vi "Lift To Inch.vi"(7 "Speed":dbl=1.0, 11 "Inches to move":dbl) -> (2 "Done":bool)   [LabVIEW 2014]
uses:
  Begin/Global Variables.vi
  <vilib>/Rock Robotics/Network Tables/SD Write Boolean.vi
  Begin/Global RefNums.vi
  <vilib>/Rock Robotics/Network Tables/SD Write Number.vi
panel:
  in  "slave offset":dbl=600.0
  in  "right PID gains":T1={"proportional gain (Kc)"=0.00225, "integral time (Ti, min)"=0.0, "derivative time (Td, min)"=0.0003} {"derivative time (Td, min)" format="%.4f"; "integral time (Ti, min)" format="%.6f"; "proportional gain (Kc)" format="%.5f"}
  in  "left PID gains":T2={"proportional gain (Kc)"=0.003, "integral time (Ti, min)"=0.0, "derivative time (Td, min)"=0.0005} {"derivative time (Td, min)" format="%.10f"; "proportional gain (Kc)" format="%.5f"}
  in  "Output Range":cluster{"output high":dbl, "output low":dbl}={"output high"=0.5, "output low"=-0.5} {"output low" format="%.2f"; "output high" format="%.2f"}
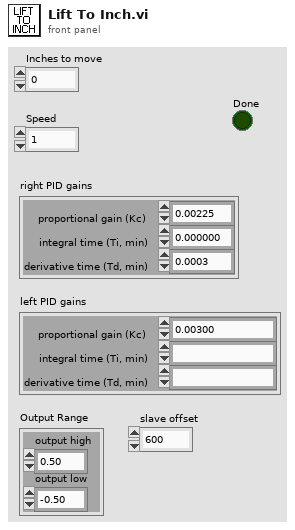
[diagram p1: front panel]
types:
  T1 = cluster{"proportional gain (Kc)":dbl, "integral time (Ti, min)":dbl, "derivative time (Td, min)":dbl}
  T2 = cluster{"proportional gain (Kc)":dbl, "integral time (Ti, min)":fxp<+/-,64,32>, "derivative time (Td, min)":dbl}
  T3 = typedef "WPI_EncoderDevRef.ctl" = cluster{"DevStatus":errorcluster, "EncoderIndex":T4, "CounterIndex":T5, "DistancePerCount":dbl, "Decoding Type":T6}
  T4 = typedef "FPGA_EncoderIdx.ctl" = enum8{"Enc 0", "Enc 1", "Enc 2", "Enc 3", "Enc 4", "Enc 5", "Enc 6", "Enc 7", "Invalid"}
  T5 = typedef "FPGA_CounterCtrSystemIndex.ctl" = enum8{"Ctr 0", "Ctr 1", "Ctr 2", "Ctr 3", "Ctr 4", "Ctr 5", "Ctr 6", "Ctr 7", "Invalid"}
  T6 = typedef "WPI_EncoderType.ctl" = enum16{"1x", "2x", "4x"}
  T7 = typedef "WPI_MotorControlDeviceRef.ctl" = cluster{"DeviceStatus":errorcluster, "Type":T8, "PWM":cluster{"Controller":T9, "PWM Channel":T10, "DeadBand":T11}, "CAN":cluster{"Device Number":u8, "Control Mode":T12, "Semaphore":T13, "Max Vout":dbl, "TalonSRX Control Mode":T14}, "Invert":bool, "TransformRef":T15, "InvTransformRef":T15}
  T8 = typedef "WPI_MotorControlType.ctl" = enum16{"PWM", "CAN", "CANTalonSRX"}
  T9 = typedef "FPGA_TypedefDigitalModule.ctl" = enum16{"Controller 1"}
  T10 = typedef "FPGA_DIOPWMChannel.ctl" = enum8{"PWM 0", "PWM 1", "PWM 2", "PWM 3", "PWM 4", "PWM 5", "PWM 6", "PWM 7", "PWM 8", "PWM 9", "PWM MXP 0", "PWM MXP 1", "PWM MXP 2", "PWM MXP 3", "PWM MXP 4", "PWM MXP 5", "PWM MXP 6", "PWM MXP 7", "PWM MXP 8", "PWM MXP 9", "Invalid"}
  T11 = typedef "WPI_PWMDeadband.ctl" = cluster{"Name":string, "maxPositivePwm":i32, "minPositivePwm":i32, "centerPwm":i32, "maxNegativePwm":i32, "minNegativePwm":i32, "angularRange":u16}
  T12 = typedef "WPI_CANJaguar_ControlMode.ctl" = enum8{"Percent VBus", "Current", "Speed", "Position", "Voltage"}
  T13 = typedef "Semaphore RefNum" = refnum<k1>
  T14 = typedef "WPI_CANTalonSRX_APIControlMode.ctl" = enum8{"Percent VBus", "Speed", "Position", "Slave", "Unchanged / Invalid"}
  T15 = typedef "WPI_PWMTransform_ConPane.ctl" = refnum<vi>
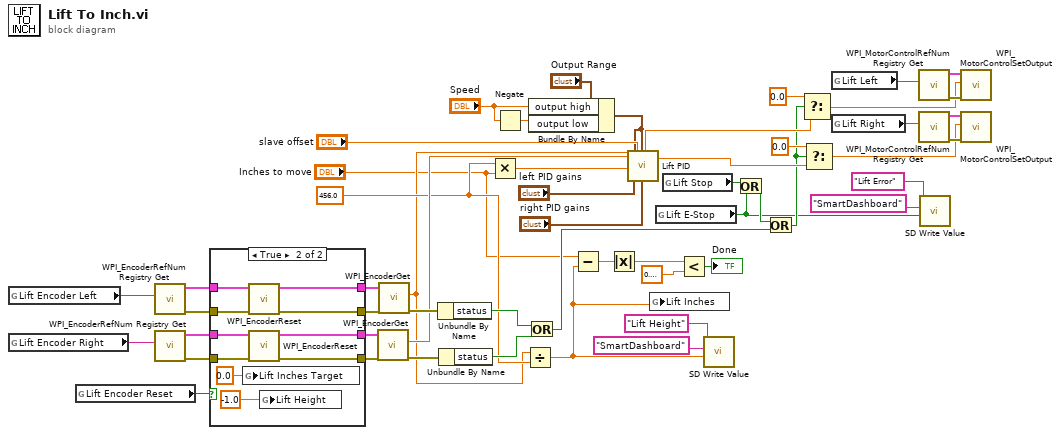
[diagram p0: block diagram]
diagram:
  w4 = 456.0 ("y")
  n1 = global read "Global RefNums.vi" "Lift Encoder Left"() -> (w14:string)
  n2 = global read "Global RefNums.vi" "Lift Encoder Right"() -> (w13:string)
  n3 = global read "Global Variables.vi" "Lift Encoder Reset"() -> (w3:bool)
  n4 = call <vilib>:"WPI_EncoderRefNum Registry Get.vi"("refnum name"=w14) -> ("error out"=w48:errorcluster, "EncoderDevRef"=w47:T3)  [unwired: 9 in]
  n5 = call <vilib>:"WPI_EncoderRefNum Registry Get.vi"("refnum name"=w13) -> ("error out"=w45:errorcluster, "EncoderDevRef"=w46:T3)  [unwired: 9 in]
  n6 = case shown="True" w3 {
    tunnel: w45 -> [w54 w67]
    tunnel: w46 -> [w55 w66]
    tunnel: w48 -> [w56 w64]
    tunnel: w47 -> [w57 w65]
    tunnel: [w57 w63] -> w50
    tunnel: [w55 w62] -> w51
    tunnel: [w54 w61] -> w52
    tunnel: [w56 w60] -> w53
    frame False {
    }
    frame True {
      n7 = global write "Global Variables.vi" "Lift Inches Target"(0.0 ("Lift Inches Target")) -> ()
      n8 = call <vilib>:"WPI_EncoderReset.vi"("error in (no error)"=w64, "EncoderDevRef"=w65) -> ("error out"=w60:errorcluster, "EncoderDevRef"=w63:T3)  [unwired: 8 in]
      n9 = call <vilib>:"WPI_EncoderReset.vi"("error in (no error)"=w67, "EncoderDevRef"=w66) -> ("error out"=w61:errorcluster, "EncoderDevRef"=w62:T3)  [unwired: 8 in]
      n10 = global write "Global Variables.vi" "Lift Height"(-1.0 ("Lift Inches Target")) -> ()
    }
  }
  n11 = call <vilib>:"WPI_EncoderGet.vi"("error in (no error)"=w52, "EncoderDevRef"=w51) -> ("error out"=w20:errorcluster, "Distance"=w11:dbl)  [unwired: 4 in, 4 out]
  n12 = call <vilib>:"WPI_EncoderGet.vi"("error in (no error)"=w53, "EncoderDevRef"=w50) -> ("error out"=w23:errorcluster, "Distance"=w2:dbl)  [unwired: 4 in, 4 out]
  n13 = Unbundle By Name(w23) -> ("status"=w21:bool)
  n14 = Unbundle By Name(w20) -> ("status"=w19:bool)
  n15 = Multiply(x=w4, y="Inches to move") -> (x*y=w34:dbl)
  n16 = Negate(x="Speed") -> (-x=w36:dbl)
  n17 = Divide(x=w2, y=w4) -> (x/y=w8:dbl)
  n18 = Or(x=w21, y=w19) -> (x .or. y?=w18:bool)
  n19 = Bundle By Name(cluster="Output Range", "output high"="Speed", "output low"=w36) -> (w37:cluster{"output high":dbl, "output low":dbl})
  n20 = Subtract(x="Inches to move", y=w8) -> (x-y=w33:dbl)
  n21 = Absolute Value(x=w33) -> (abs(x)=w32:dbl)
  n22 = call "Lift PID.vi"("left encoder"=w2, "right encoder"=w11, "move to distance"=w34, "left output range"=w37, "left PID gains"="left PID gains", "slave offset"="slave offset", "right output range"=w37, "right PID gains"="right PID gains") -> ("lift motor left"=w24:dbl, "lift motor right"=w25:dbl)  [unwired: 18 in]
  n23 = global write "Global Variables.vi" "Lift Inches"(w8) -> ()
  n24 = global read "Global Variables.vi" "Lift E-Stop"() -> (w5:bool)
  n25 = global read "Global Variables.vi" "Lift Stop"() -> (w12:bool)
  n26 = Less?(x=w32, y=0.20000000000000004) -> (x < y?=→"Done":bool)
  n27 = call-poly <vilib>:"SD Write Value.vi"("Numeric"=w8, "Table Prefix"="SmartDashboard", "Name"="Lift Height") -> ()  [unwired: 7 in, 2 out]
  n28 = Or(x=w12, y=w5) -> (x .or. y?=w17:bool)
  n29 = Or(x=w17, y=w18) -> (x .or. y?=w22:bool)
  n30 = Select(t=0.0, s=w22, f=w24) -> (s? t:f=w27:dbl)
  n31 = Select(t=0.0, s=w22, f=w25) -> (s? t:f=w26:dbl)
  n32 = global read "Global RefNums.vi" "Lift Left"() -> (w16:string)
  n33 = global read "Global RefNums.vi" "Lift Right"() -> (w15:string)
  n34 = call <vilib>:"WPI_MotorControlRefNum Registry Get.vi"("refnum name"=w16) -> ("error out"=w42:errorcluster, "MotorControlDevRef"=w41:T7)  [unwired: 9 in]
  n35 = call <vilib>:"WPI_MotorControlRefNum Registry Get.vi"("refnum name"=w15) -> ("error out"=w39:errorcluster, "MotorControlDevRef"=w40:T7)  [unwired: 9 in]
  n36 = call-poly <vilib>:"SD Write Value.vi"("Boolean"=w5, "Table Prefix"="SmartDashboard", "Name"="Lift Error") -> ()  [unwired: 7 in, 2 out]
  n37 = call <vilib>:"WPI_MotorControlSetOutput.vi"("error in (no error)"=w42, "Output"=w27, "MotorControlDevRef"=w41) -> ()  [unwired: 6 in, 3 out]
  n38 = call <vilib>:"WPI_MotorControlSetOutput.vi"("error in (no error)"=w39, "Output"=w26, "MotorControlDevRef"=w40) -> ()  [unwired: 6 in, 3 out]
